vi "SetSystemParameterFloat.vi"(6 "error in (no error)":errorcluster, 7 "value":sgl, 8 "Parameter Name":string(combo), 9 "controller in":refnum<k24>) -> (0 "error out":errorcluster, 3 "controller out":refnum<k24>)   [LabVIEW 2013]
uses:
  C:/GEECS/Developers Version/source/Device Driver/AerotechStage/Sample Vis/Bin/Aerotech.Ensemble.dll
  Bin/Aerotech.Ensemble.dll
  C:/GEECS/Developers Version/source/Device Driver/AerotechStage/Sample Vis/Bin/Aerotech.Ensemble.LabVIEW.dll
  Bin/Aerotech.Ensemble.LabVIEW.dll
panel:
  out "ParameterType":i32(ring)=2 items=["Integer", "Double", "Single", "Long", "String"]
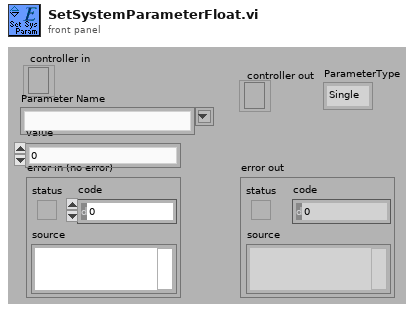
[diagram p1: front panel]
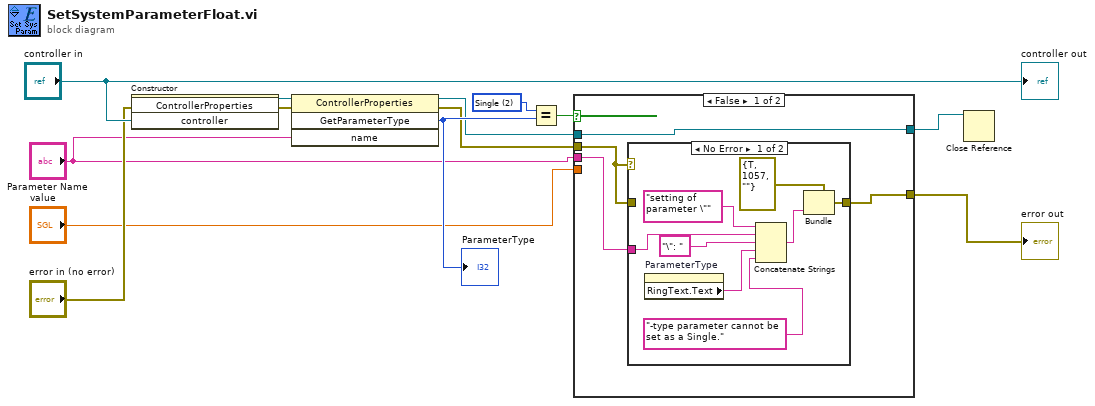
[diagram p0: block diagram]
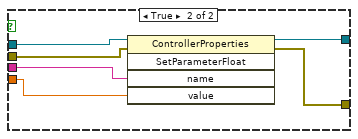
[diagram p3: hidden frame]
diagram:
  w9 = 2 items=["Integer", "Double", "Single", "Long", "String"] ("GetParameterType")
  n1 = constructor class="ControllerProperties"(error in="error in (no error)", "controller"="controller in") -> (reference out=w11:refnum<k24>, error out=w10:errorcluster)  [unwired: 2 in, 2 out]
  n2 = invoke class="ControllerProperties" method="GetParameterType"(reference=w11, error in=w10, "name"="Parameter Name") -> (reference out=w5:refnum<k24>, error out=w4:errorcluster, "GetParameterType"=w8:i32)  [unwired: 1 in, 1 out]
  "ParameterType" <- w8
  n3 = Equal?(x=w9, y=w8) -> (x = y?=w7:bool)
  n4 = case shown="False" w7 {
    tunnel: [w17 w31] -> w6
    tunnel: w5 -> [w17 w32]
    tunnel: "Parameter Name" -> [w14 w30]
    tunnel: w4 -> [w15 w29]
    tunnel: [w16 w28] -> w3
    tunnel: "value" -> [_ w27]
    frame False {
      n5 = case shown="No Error" w15 {
        tunnel: [w24 w26] -> w16
        tunnel: w15 -> [_ w26]
        tunnel: w14 -> [w21 _]
        frame No Error {
          n6 = property on="ParameterType" class="Ring (strict)"() -> ("RingText.Text"=w19:string)  [unwired: 2 in, 2 out]
          n7 = Concatenate Strings("setting of parameter \"" ("string"), w21, "\": " ("string"), w19, "-type parameter cannot be set as a Single." ("string")) -> (w23:string)
          n8 = Bundle(cluster=cluster{bool, "code":i32, "source":string} {TRUE, "code"=1057, "source"=""} ("error out"), "source"=w23) -> (w24:cluster{bool, "code":i32, "source":string})  [unwired: 2 in]
        }
        frame Error {
        }
      }
    }
    frame True {
      n9 = invoke class="ControllerProperties" method="SetParameterFloat"(reference=w32, error in=w29, "name"=w30, "value"=w27) -> (reference out=w31:refnum<k24>, error out=w28:errorcluster)  [unwired: 1 in, 3 out]
    }
  }
  "error out" <- w3
  n10 = Close Reference(reference=w6) -> ()  [unwired: 1 in, 1 out]
  "controller out" <- "controller in"
